vi "Initialization VI.vi"(8 "error in (no error)":errorcluster, 10 "Custom XML":string, 11 "Device Item Ref in":T2 format="%.0x") -> (0 "error out":errorcluster, 3 "Device Item Ref out":T2 format="%.0x")   [LabVIEW 2010]
uses:
  <vilib>/NI Veristand/Custom Device API/Custom Device API.lvlib
  <vilib>/NI VeriStand/Custom Device API/Custom Device Channel Type.ctl
  <vilib>/NI VeriStand/Custom Device API/Custom Device Channel.ctl
  <vilib>/NI VeriStand/Custom Device API/Custom Device Loop Type.ctl
  <vilib>/NI VeriStand/Custom Device API/Custom Device Item Ref.ctl
  Channel Data.ctl
panel:
  in  "Channel Data (DBLs Only)":T1
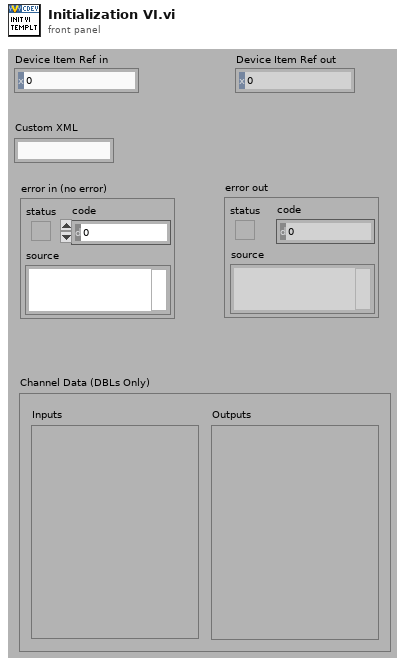
[diagram p1: front panel]
types:
  T1 = typedef "Channel Data.ctl" = cluster{"Inputs":cluster{}, "Outputs":cluster{}}
  T2 = typedef "Custom Device API.lvlib/Custom Device Item Ref.ctl" = u64
  T3 = typedef "Custom Device API.lvlib/Custom Device Loop Type.ctl" = enum32{"While Loop", "Timed Loop"}
  T4 = typedef "Custom Device API.lvlib/Custom Device Channel.ctl" = cluster{"Type":T5, "Units":string, "Default Value":dbl, "Faultable":bool, "Scalable":bool}
  T5 = typedef "Custom Device API.lvlib/Custom Device Channel Type.ctl" = enum16{"Input", "Output"}
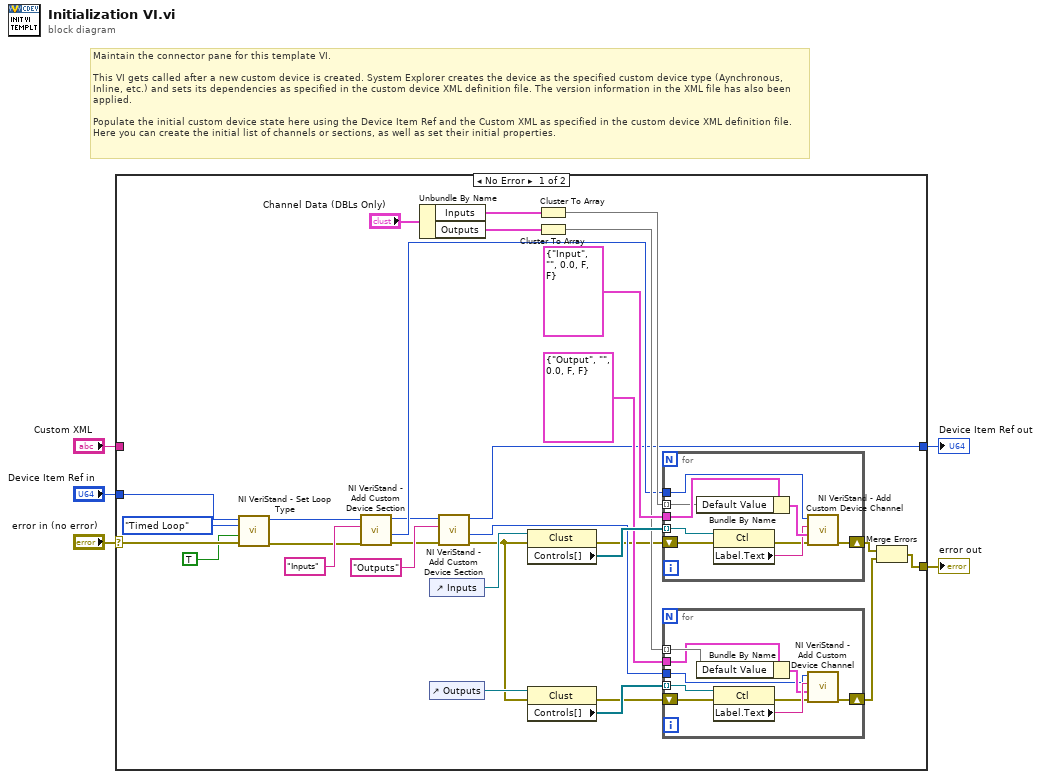
[diagram p0: block diagram]
diagram:
  # "Maintain the connector pane for this template VI.\n\nThis VI gets called after a new custom device is created. System Explorer creates the device as the specified custom device type (Aynchronous, Inline, etc.) and sets its dependencies as specified in the custom device XML definition file. The version information in the XML file has also been applied.\n\nPopulate the initial custom device state here using the Device Item Ref and the Custom XML as specified in the custom device XML definition file. Here you can create the initial list of channels or sections, as well as set their initial properties."
  n1 = case shown="No Error" "error in (no error)" {
    selector: "error in (no error)" -> [w11 w55]
    tunnel: [w14 w55] -> w5
    tunnel: [w19 w54] -> w3
    tunnel: "Device Item Ref in" -> [w9 w54]
    tunnel: "Custom XML" -> [_ _]
    frame No Error {
      n2 = call <vilib>:"NI VeriStand - Set Loop Type.vi"("error in (no error)"=w11, "Use Device Clock (Timed Loops only)"=TRUE, "Loop type"=Custom_Device_Loop_Type."Timed Loop", "Device Ref in"=w9) -> ("error out"=w10:errorcluster, "Device Ref out"=w8:T2)  [unwired: 6 in]
      n3 = call <vilib>:"NI VeriStand - Add Custom Device Section.vi"("error in (no error)"=w10, "Section Name"="Inputs", "Parent Ref in"=w8) -> ("error out"=w18:errorcluster, "Section Ptr"=w23:T2, "Parent Ref out"=w22:T2)  [unwired: 5 in, 1 out]
      n4 = Unbundle By Name("Channel Data (DBLs Only)") -> ("Inputs"=w33:cluster{}, "Outputs"=w26:cluster{})
      n5 = control-ref of="Inputs"() -> (w31:refnum<vi>)
      n6 = control-ref of="Outputs"() -> (w28:refnum<vi>)
      n7 = call <vilib>:"NI VeriStand - Add Custom Device Section.vi"("error in (no error)"=w18, "Section Name"="Outputs", "Parent Ref in"=w22) -> ("error out"=w17:errorcluster, "Section Ptr"=w20:T2, "Parent Ref out"=w19:T2)  [unwired: 5 in, 1 out]
      n8 = property class="Clust"(reference=w31, error in=w17) -> (error out=w13:errorcluster, "Controls[]"=w30:refnum<vi>[])  [unwired: 1 out]
      n9 = property class="Clust"(reference=w28, error in=w17) -> (error out=w12:errorcluster, "Controls[]"=w27:refnum<vi>[])  [unwired: 1 out]
      n10 = Cluster To Array(cluster=w33) -> (array=w29:void[])
      n11 = Cluster To Array(cluster=w26) -> (array=w25:void[])
      n12 = for {
        tunnel: w29 -> [w50] mode=indexing
        tunnel: T4 {"Type"=enum."Input", "Units"="", "Default Value"=0.0, "Faultable"=FALSE, "Scalable"=FALSE} ("Channel") -> [w51]
        tunnel: w23 -> [w53]
        tunnel: w30 -> [w52] mode=indexing
        shift-right: [w47] -> w16
        shift-left: w13 -> [w46]
        n13 = Bundle By Name(cluster=w51, "Default Value"=w50) -> (w49:T4)
        n14 = property class="Ctl"(reference=w52, error in=w46) -> (error out=w45:errorcluster, "Label.Text"=w48:string)  [unwired: 1 out]
        n15 = call <vilib>:"NI VeriStand - Add Custom Device Channel.vi"("error in (no error)"=w45, "Channel"=w49, "Channel Name"=w48, "Parent Ref in"=w53) -> ("error out"=w47:errorcluster)  [unwired: 4 in, 3 out]
      }
      n16 = for {
        tunnel: w27 -> [w43] mode=indexing
        tunnel: w25 -> [w42] mode=indexing
        tunnel: T4 {"Type"=enum."Output", "Units"="", "Default Value"=0.0, "Faultable"=FALSE, "Scalable"=FALSE} ("Channel") -> [w41]
        tunnel: w20 -> [w39]
        shift-right: [w37] -> w15
        shift-left: w12 -> [w36]
        n17 = Bundle By Name(cluster=w41, "Default Value"=w42) -> (w40:T4)
        n18 = property class="Ctl"(reference=w43, error in=w36) -> (error out=w38:errorcluster, "Label.Text"=w44:string)  [unwired: 1 out]
        n19 = call <vilib>:"NI VeriStand - Add Custom Device Channel.vi"("error in (no error)"=w38, "Channel"=w40, "Channel Name"=w44, "Parent Ref in"=w39) -> ("error out"=w37:errorcluster)  [unwired: 4 in, 3 out]
      }
      n20 = Merge Errors(w16, w15) -> (w14:errorcluster)
    }
    frame Error {
    }
  }
  "error out" <- w5
  "Device Item Ref out" <- w3
